vi "fit magnet to position.vi"(5 "triggered?":bool=TRUE, 7 "graph type":T2(ring), 8 "error in (no error)":errorcluster, 9 "crossing-2":dbl=-inf, 10 "current crossing":dbl=inf, 11 "display queues":T3) -> (0 "error out":errorcluster, 1 "angle and time":T1, 2 "mag time graphs":cluster{dbl[], "best nonlinear fit":dbl[]}[](array[cluster]), 3 "mag xy position":cluster{dbl[], dbl[]}[](array[cluster]), 4 "mag pos axes limits":cluster{"mag pos max":dbl, "mag pos min":dbl}, 6 "fit parameters":cluster{"a":dbl, "b":dbl, "theta":dbl, "b0":dbl})   [LabVIEW 2017]
uses:
  typedefs/queue cluster.ctl
  typedefs/reading queue.ctl
  typedefs/reading.ctl
  typedefs/readingType.ctl
  typedefs/reading 1 queue.ctl
  typedefs/reading1.ctl
  <vilib>/Analysis/baseanly.llb/Mean (DBL).vi
  <vilib>/gmath/NumericalOptimization/Nonlinear Curve Fit LM formula string.vi
  <vilib>/gmath/NI_Gmath.lvlib
  <vilib>/Analysis/NI_AALBase.lvlib
panel:
  out "fitter error":bool
  out "rparallel":dbl[](array[numeric])
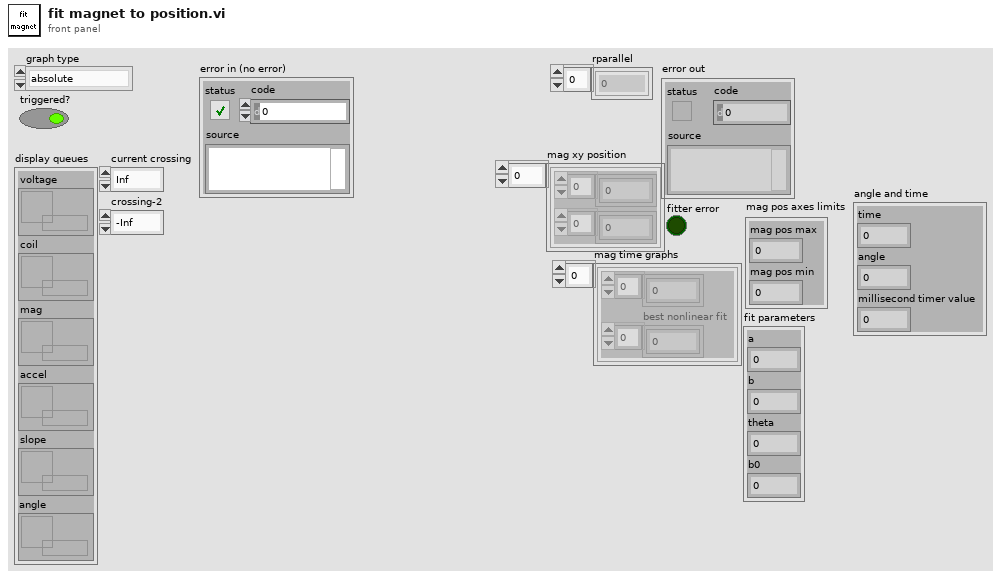
[diagram p1: front panel]
types:
  T1 = cluster{"time":dbl, "angle":dbl, "millisecond timer value":u32}
  T2 = enum16{"absolute", "relative", "positional", "position only"}
  T3 = typedef "queue cluster.ctl" = cluster{"voltage":T4, "coil":T4, "mag":T4, "accel":T4, "slope":T5, "angle":T4}
  T4 = typedef "reading queue.ctl" = refnum<queue>
  T5 = typedef "reading 1 queue.ctl" = refnum<queue>
  T6 = cluster{"model":string, "Parameters":string[], "x":string}
  T7 = typedef "reading.ctl" = cluster{"reading type":T8, "time":fxp<+,48,48>, "x":sgl, "y":sgl, "z":sgl, "XSUM":u8}
  T8 = typedef "readingType.ctl" = enum8{"SYNC", "DETVAL", "COILI", "MAGVEC", "ACCVEC"}
  T9 = cluster{"Best Linear Fit":dbl[], "Best Linear Fit":dbl[]}[]
  T10 = cluster{"mean":dbl, "angle":dbl, "millisecond timer value":u32}
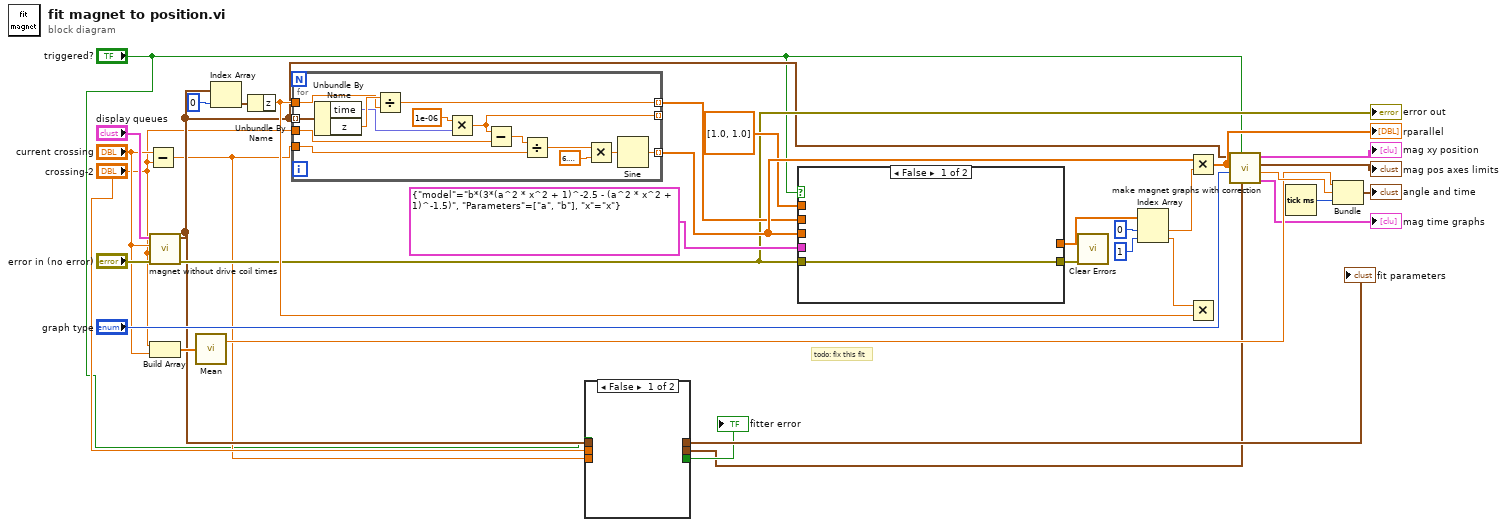
[diagram p0: block diagram]
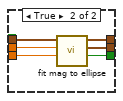
[diagram p2: hidden frame]
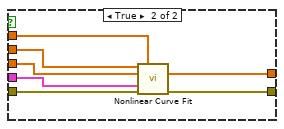
[diagram p3: hidden frame]
diagram:
  # "todo: fix this fit"
  n1 = Subtract(x="current crossing", y="crossing-2") -> (x-y=w5:dbl)
  n2 = call "magnet without drive coil times.vi"("error in (no error)"="error in (no error)", "min time"="crossing-2", "max time"="current crossing", "display queues"="display queues") -> ("error out"=w9:errorcluster, "mag no drive"=w7:T7[])  [unwired: 5 in, 1 out]
  "error out" <- w9
  n3 = Build Array("crossing-2", "current crossing") -> (w16:dbl[])
  n4 = call-poly <vilib>:"Mean.vi"("X"=w16) -> ("mean"=w13:dbl)  [unwired: 1 out]
  n5 = Index Array(array=w7, index=0) -> (element=w33:T7)
  n6 = Unbundle By Name(w33) -> ("z"=w24:sgl)
  n7 = for {
    tunnel: w7 -> [w48] mode=indexing
    tunnel: w5 -> [w45]
    tunnel: "crossing-2" -> [w47]
    tunnel: [w38] -> w28 mode=indexing
    tunnel: w24 -> [w41]
    tunnel: [w40] -> w22 mode=indexing
    tunnel: [w36] -> _ mode=indexing
    n8 = Unbundle By Name(w48) -> ("time"=w37:fxp<+,48,48>, "z"=w42:sgl)
    n9 = Divide(x=w42, y=w41) -> (x/y=w40:sgl)
    n10 = Multiply(x=1e-06, y=w37) -> (x*y=w36:dbl)
    n11 = Subtract(x=w36, y=w47) -> (x-y=w46:dbl)
    n12 = Divide(x=w46, y=w45) -> (x/y=w44:dbl)
    n13 = Multiply(x=w44, y=6.283185307179586) -> (x*y=w39:dbl)
    n14 = Sine(x=w39) -> (sin(x)=w38:dbl)
  }
  n15 = case shown="False" "triggered?" {
    tunnel: w7 -> [_ w54]
    tunnel: "crossing-2" -> [_ w53]
    tunnel: w5 -> [_ w52]
    tunnel: [_ w51] -> w4
    tunnel: [_ w50] -> w3
    tunnel: [_ w49] -> w2
    frame False {
    }
    frame True {
      n16 = call "fit mag to ellipse.vi"("T"=w52, "t0"=w53, "mag no drive"=w54) -> ("fitter error"=w50:bool, "fit magnetic field"=w49:T7[], "fit parameters"=w51:cluster{"a":dbl, "b":dbl, "theta":dbl, "b0":dbl})  [unwired: 6 in]
    }
  }
  "fit parameters" <- w4
  "fitter error" <- w3
  n17 = case shown="False" "triggered?" {
    tunnel: T6 {"model"="b*(3*(a^2 * x^2 + 1)^-2.5 - (a^2 * x^2 + 1)^-1.5)", "Parameters"=["a", "b"], "x"="x"} ("model description") -> [_ w62]
    tunnel: [_ w61] -> w30
    tunnel: w28 -> [_ w60]
    tunnel: dbl[] [1.0, 1.0] ("initial parameters") -> [_ w59]
    tunnel: w22 -> [_ w58]
    tunnel: [w55 w57] -> w20
    tunnel: w9 -> [w55 w56]
    frame False {
    }
    frame True {
      n18 = call-poly <vilib>:"Nonlinear Curve Fit.vi"("Y"=w58, "initial parameters"=w59, "X"=w60, "model description"=w62, "error in (no error)"=w56) -> ("best fit parameters"=w61:dbl[], "error out"=w57:errorcluster)  [unwired: 6 in, 3 out]
    }
  }
  n19 = call <vilib>:"Clear Errors.vi"("error in (no error)"=w20) -> ()  [unwired: 5 in, 2 out]
  n20 = Index Array(array=w30, index #1=0 ("index"), index #2=1 ("index")) -> (element #1=w29:dbl, element #2=w25:dbl)
  n21 = Multiply(x=w28, y=w29) -> (x*y=w19:dbl[])
  "rparallel" <- w19
  n22 = Multiply(x=w25, y=w24) -> ()  [unwired: 1 out]
  n23 = call "make magnet graphs with correction.vi"("fit magnetic field"=w2, "triggered?"="triggered?", "graph type"="graph type", "rbar_parallel"=w19, "mag no drive"=w7) -> ("mag time graphs"=→"mag time graphs":cluster{dbl[], dbl[]}[], "angle"=w15:dbl, "mag pos axes limits"=→"mag pos axes limits":cluster{"mag pos max":dbl, "mag pos min":dbl}, "mag position graphs"=→"mag xy position":T9)  [unwired: 2 in, 1 out]
  n24 = Tick Count (ms)() -> (millisecond timer value=w14:u32)
  n25 = Bundle("mean"=w13, "angle"=w15, "millisecond timer value"=w14) -> (→"angle and time":T10)  [unwired: 1 in]
